vi "Abort.vi"(8 "error in (no error)":errorcluster, 10 "Sequence Name":string, 11 "Sequencing in":refnum<class "Sequencing.lvclass">) -> (0 "error out":errorcluster, 3 "Sequencing out":refnum<class "Sequencing.lvclass">)   [LabVIEW 2020, in "VolatusSeq.lvlib" / "Sequencing.lvclass"]
uses:
  Sequencing.lvclass
  Sequencing.lvclass/Sequencing.ctl
  Sequence/Sequence.lvclass
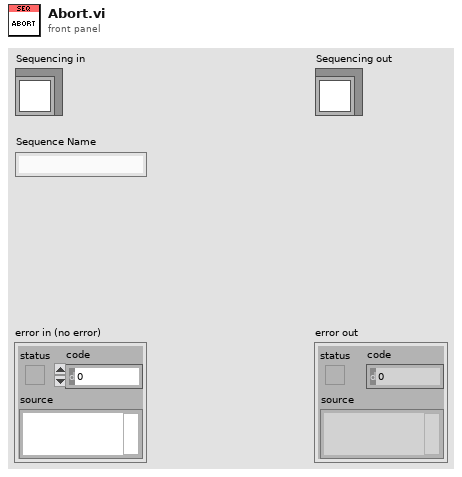
[diagram p1: front panel]
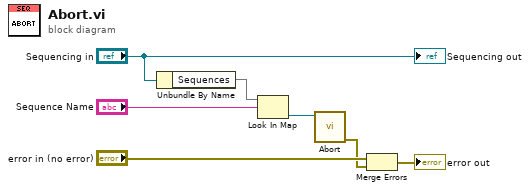
[diagram p0: block diagram]
diagram:
  n1 = Unbundle By Name("Sequencing in") -> ("Sequences"=w5:map{string, refnum<class "Sequence.lvclass">})
  n2 = Look In Map(map=w5, key="Sequence Name") -> (value=w3:refnum<class "Sequence.lvclass">)  [unwired: 1 in, 1 out]
  n3 = call "Abort.vi"("Sequence in"=w3) -> ("error out"=w1:errorcluster)  [unwired: 9 in, 1 out]
  n4 = Merge Errors("error in (no error)", w1) -> (→"error out":errorcluster)
  "Sequencing out" <- "Sequencing in"
